vi "LED Set Modes.vi"() -> ()   [LabVIEW 2017]
uses:
  LED Control Type.ctl
  LED Globals.vi
  Intake/Intake Globals.vi
panel:
  out "error out 2":errorcluster
  out "error out":errorcluster
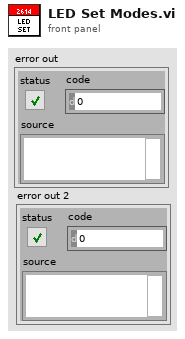
[diagram p1: front panel]
types:
  T1 = typedef "LED Control Type.ctl" = enum16{"Off", "Waiting On Field", "Connected ", "Cube In Intake", "Climbing", "Auto Cube Capture", "Ready for Cube Floor", "Ready for Cube Portal"}
  T2 = typedef "LED Notifier.ctl" = cluster{"LED Control Type":T1, "Climbing":bool, "Auto Tracking":bool, "Ready for Cube Floor":bool, "Ready for Cube Portal":bool}
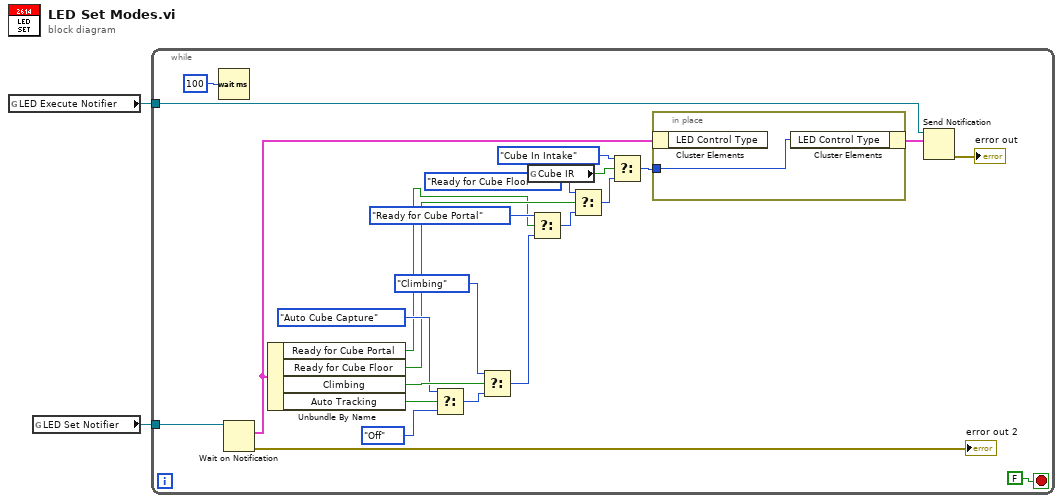
[diagram p0: block diagram]
diagram:
  n1 = global read "LED Globals.vi" "LED Execute Notifier"() -> (w1:refnum<notifier>)
  n2 = global read "LED Globals.vi" "LED Set Notifier"() -> (w2:refnum<notifier>)
  n3 = while {
    tunnel: w2 -> [w23]
    tunnel: w1 -> [w22]
    stop <- FALSE stop-if-true
    n4 = Wait (ms)(milliseconds to wait=u32 100) -> ()  [unwired: 1 out]
    n5 = Wait on Notification(notifier=w23) -> (notification=w13:T2, error out=→"error out 2":errorcluster)  [unwired: 3 in, 2 out]
    n6 = Unbundle By Name(w13) -> ("Ready for Cube Portal"=w4:bool, "Ready for Cube Floor"=w9:bool, "Climbing"=w19:bool, "Auto Tracking"=w16:bool)
    n7 = Select(t=LED_Control_Type."Auto Cube Capture" ("LED Control Type"), s=w16, f=LED_Control_Type."Off") -> (s? t:f=w17:T1)
    n8 = Select(t=LED_Control_Type."Climbing" ("LED Control Type"), s=w19, f=w17) -> (s? t:f=w18:T1)
    n9 = global read "Intake Globals.vi" "Cube IR"() -> (w3:bool)
    n10 = Select(t=LED_Control_Type."Ready for Cube Portal" ("LED Control Type"), s=w4, f=w18) -> (s? t:f=w10:T1)
    n11 = Select(t=LED_Control_Type."Ready for Cube Floor" ("LED Control Type"), s=w9, f=w10) -> (s? t:f=w7:T1)
    n12 = Select(t=LED_Control_Type."Cube In Intake" ("LED Control Type"), s=w3, f=w7) -> (s? t:f=w6:T1)
    n13 = in-place {
      in-place-border: w6 -> [w27]
      n14 = in-place-cluster #1(w13) -> ()  [unwired: 1 out]
      n15 = in-place-cluster #1("LED Control Type"=w27) -> (w24:T2)
    }
    n16 = Send Notification(notification=w24, notifier=w22) -> (error out=→"error out":errorcluster)  [unwired: 1 in, 1 out]
  }
